vi "solar_voy_def Variant Create.vi"(8 "error in (no error)":errorcluster, 9 "Enum Names":string[](array[string]), 10 "Name":string, 11 "LVTYPE":T1) -> (0 "error out":errorcluster, 3 "Variant":variant)   [LabVIEW 2018]
doc: "This VI returns the data type of the variant. Not all data types are supported. Array of clusters are not supported."
uses:
  <vilib>/Utility/Data Type/NI_Data Type.lvlib
  <vilib>/Utility/Data Type/Type Definitions/Memory Type.ctl
  <vilib>/Utility/Data Type/Type Definitions/Memory Info.ctl
  type/solar_type Item Type.ctl
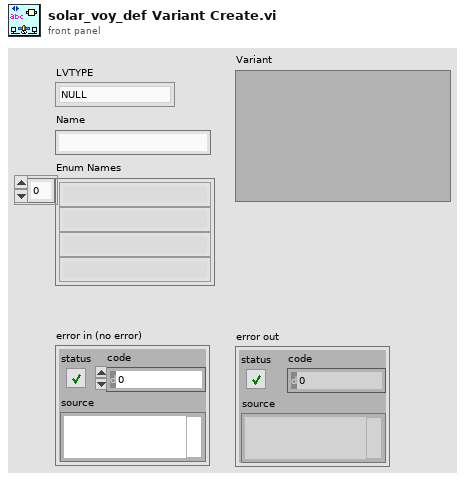
[diagram p1: front panel]
types:
  T1 = typedef "solar_type Item Type.ctl" = enum16{"NULL", "UNKNOWN", "CLUSTER", "I8", "I16", "I32", "I64", "U8", "U16", "U32", "U64", "U8_ENUM", "U16_ENUM", "U32_ENUM", "SGL", "DBL", "BOOLEAN", "STRING", "PATH", "VISA", "TAG", "TIME", "I8_1D", "I16_1D", "I32_1D", "I64_1D", "U8_1D", "U16_1D", "U32_1D", "U64_1D", "U8_ENUM_1D", "U16_ENUM_1D", "U32_ENUM_1D", "SGL_1D", "DBL_1D", "BOOLEAN_1D", "STRING_1D", "PATH_1D", "VISA_1D", "TAG_1D", "TIME_1D", "I8_2D", "I16_2D", "I32_2D", "I64_2D", "U8_2D", "U16_2D", "U32_2D", "U64_2D", "U8_ENUM_2D", "U16_ENUM_2D", "U32_ENUM_2D", "SGL_2D", "DBL_2D", "BOOLEAN_2D", "STRING_2D", "PATH_2D", "VISA_2D", "TAG_2D", "TIME_2D"}
  T2 = typedef "NI_Data Type.lvlib/Memory Info.ctl" = cluster{"Type":T3, "Size":u32}
  T3 = typedef "NI_Data Type.lvlib/Memory Type.ctl" = enum16{"Variable", "Fixed", "Bounded"}
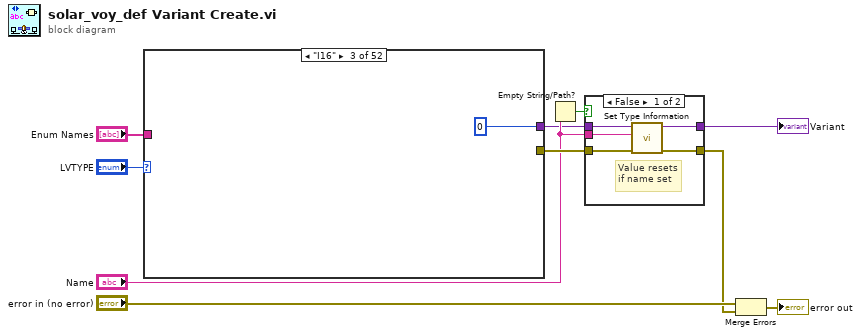
[diagram p0: block diagram]
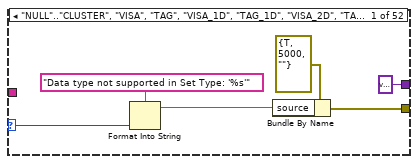
[diagram p3: hidden frame]
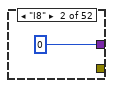
[diagram p4: hidden frame]
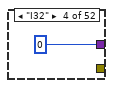
[diagram p5: hidden frame]
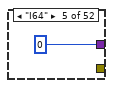
[diagram p6: hidden frame]
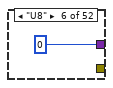
[diagram p7: hidden frame]
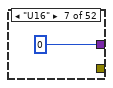
[diagram p8: hidden frame]
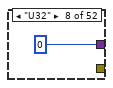
[diagram p9: hidden frame]
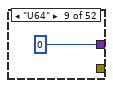
[diagram p10: hidden frame]
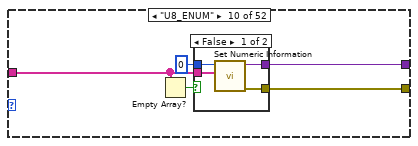
[diagram p11: hidden frame]
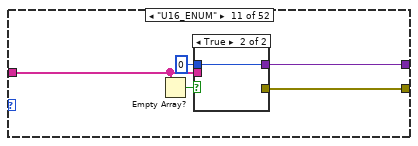
[diagram p13: hidden frame]
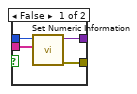
[diagram p14: hidden frame]
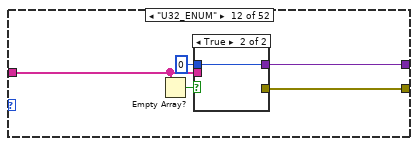
[diagram p15: hidden frame]
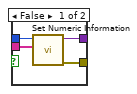
[diagram p16: hidden frame]
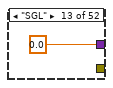
[diagram p17: hidden frame]
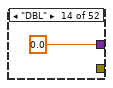
[diagram p18: hidden frame]
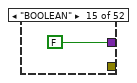
[diagram p19: hidden frame]
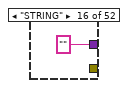
[diagram p20: hidden frame]
diagram:
  n1 = case shown="\"I16\"" "LVTYPE" {
    selector: "LVTYPE" -> [w13 _ _ _ _ _ _ _ _ _ _ _ _ _ _ _ _ _ _ _ _ _ _ _ _ _ _ _ _ _ _ _ _ _ _ _ _ _ _ _ _ _ _ _ _ _ _ _ _ _ _ _]
    tunnel: [w12 _ _ _ _ _ _ _ _ w27 w37 w47 _ _ _ _ _ _ _ _ _ _ _ _ _ _ w71 w85 w99 _ _ _ _ _ _ _ _ _ _ _ _ _ _ w128 w143 w158 _ _ _ _ _ _] -> w9
    tunnel: [variant ("Variant") i8 0 i16 0 0 i64 0 u8 0 u16 0 u32 0 u64 0 w28 w38 w48 sgl 0.0 0.0 FALSE "" path "" timestamp(0 s since 1904-01-01) i8[] [] i16[] [] i32[] [] i64[] [] u8[] [] u16[] [] u32[] [] u64[] [] w70 w84 w98 sgl[] [] dbl[] [] bool[] [] string[] [] path[] [] timestamp[] [] i8[][] [] i16[][] [] i32[][] [] i64[][] [] u8[][] [] u16[][] [] u32[][] [] u64[][] [] w127 w142 w157 sgl[][] [] dbl[][] [] bool[][] [] string[][] [] path[][] [] timestamp[][] []] -> w7
    tunnel: "Enum Names" -> [_ _ _ _ _ _ _ _ _ w26 w36 w46 _ _ _ _ _ _ _ _ _ _ _ _ _ _ w69 w83 w97 _ _ _ _ _ _ _ _ _ _ _ _ _ _ w126 w141 w156 _ _ _ _ _ _]
    frame "NULL".."CLUSTER", "VISA", "TAG", "VISA_1D", "TAG_1D", "VISA_2D", "TAG_2D" {
      n2 = Format Into String(format string="Data type not supported in Set Type: '%s'" ("source"), w13) -> (resulting string=w16:string)  [unwired: 2 in, 1 out]
      n3 = Bundle By Name(cluster=errorcluster {"status"=TRUE, "code"=5000, "source"=""} ("error out"), "source"=w16) -> (w12:errorcluster)
    }
    frame "I8" {
    }
    frame "I16" {
    }
    frame "I32" {
    }
    frame "I64" {
    }
    frame "U8" {
    }
    frame "U16" {
    }
    frame "U32" {
    }
    frame "U64" {
    }
    frame "U8_ENUM" {
      n4 = Empty Array?(array=w26) -> (empty?=w25:bool)
      n5 = case shown="False" w25 {
        tunnel: u8 0 -> [w33 w34]
        tunnel: [w32 w34] -> w28
        tunnel: [w31 _] -> w27
        tunnel: w26 -> [w30 _]
        frame False {
          n6 = call <vilib>:"Set Numeric Information.vi"("Enum Names"=w30, "Variant in"=w33) -> ("error out"=w31:errorcluster, "Variant out"=w32:variant)  [unwired: 8 in]
        }
        frame True {
        }
      }
    }
    frame "U16_ENUM" {
      n7 = Empty Array?(array=w36) -> (empty?=w35:bool)
      n8 = case shown="True" w35 {
        tunnel: u16 0 -> [w43 w44]
        tunnel: [w42 w44] -> w38
        tunnel: [w41 _] -> w37
        tunnel: w36 -> [w40 _]
        frame False {
          n9 = call <vilib>:"Set Numeric Information.vi"("Enum Names"=w40, "Variant in"=w43) -> ("error out"=w41:errorcluster, "Variant out"=w42:variant)  [unwired: 8 in]
        }
        frame True {
        }
      }
    }
    frame "U32_ENUM" {
      n10 = Empty Array?(array=w46) -> (empty?=w45:bool)
      n11 = case shown="True" w45 {
        tunnel: u32 0 -> [w53 w54]
        tunnel: [w52 w54] -> w48
        tunnel: [w51 _] -> w47
        tunnel: w46 -> [w50 _]
        frame False {
          n12 = call <vilib>:"Set Numeric Information.vi"("Enum Names"=w50, "Variant in"=w53) -> ("error out"=w51:errorcluster, "Variant out"=w52:variant)  [unwired: 8 in]
        }
        frame True {
        }
      }
    }
    frame "SGL" {
    }
    frame "DBL" {
    }
    frame "BOOLEAN" {
    }
    frame "STRING" {
    }
    frame "PATH" {
    }
    frame "TIME" {
    }
    frame "I8_1D" {
    }
    frame "I16_1D" {
    }
    frame "I32_1D" {
    }
    frame "I64_1D" {
    }
    frame "U8_1D" {
    }
    frame "U16_1D" {
    }
    frame "U32_1D" {
    }
    frame "U64_1D" {
    }
    frame "U8_ENUM_1D" {
      w74 = u8[] []
      n13 = Index Array(array=w74) -> (element=w73:u8)  [unwired: 1 in]
      n14 = Empty Array?(array=w69) -> (empty?=w77:bool)
      n15 = case shown="True" w77 {
        tunnel: w73 -> [w81 w82]
        tunnel: [w80 w82] -> w76
        tunnel: [w79 _] -> w72
        tunnel: w69 -> [w78 _]
        frame False {
          n16 = call <vilib>:"Set Numeric Information.vi"("Enum Names"=w78, "Variant in"=w81) -> ("error out"=w79:errorcluster, "Variant out"=w80:variant)  [unwired: 8 in]
        }
        frame True {
        }
      }
      n17 = call <vilib>:"Set Array Information.vi"("error in (no error)"=w72, "Array Lengths"=T2[] [{"Type"=enum."Variable", "Size"=0}], "Array Element"=w76, "Variant in"=w74) -> ("error out"=w71:errorcluster, "Variant out"=w70:variant)  [unwired: 6 in]
    }
    frame "U16_ENUM_1D" {
      w88 = u16[] []
      n18 = Index Array(array=w88) -> (element=w87:u16)  [unwired: 1 in]
      n19 = Empty Array?(array=w83) -> (empty?=w91:bool)
      n20 = case shown="True" w91 {
        tunnel: w87 -> [w95 w96]
        tunnel: [w94 w96] -> w90
        tunnel: [w93 _] -> w86
        tunnel: w83 -> [w92 _]
        frame False {
          n21 = call <vilib>:"Set Numeric Information.vi"("Enum Names"=w92, "Variant in"=w95) -> ("error out"=w93:errorcluster, "Variant out"=w94:variant)  [unwired: 8 in]
        }
        frame True {
        }
      }
      n22 = call <vilib>:"Set Array Information.vi"("error in (no error)"=w86, "Array Lengths"=T2[] [{"Type"=enum."Variable", "Size"=0}], "Array Element"=w90, "Variant in"=w88) -> ("error out"=w85:errorcluster, "Variant out"=w84:variant)  [unwired: 6 in]
    }
    frame "U32_ENUM_1D" {
      w102 = u32[] []
      n23 = Index Array(array=w102) -> (element=w101:u32)  [unwired: 1 in]
      n24 = Empty Array?(array=w97) -> (empty?=w105:bool)
      n25 = case shown="True" w105 {
        tunnel: w101 -> [w109 w110]
        tunnel: [w108 w110] -> w104
        tunnel: [w107 _] -> w100
        tunnel: w97 -> [w106 _]
        frame False {
          n26 = call <vilib>:"Set Numeric Information.vi"("Enum Names"=w106, "Variant in"=w109) -> ("error out"=w107:errorcluster, "Variant out"=w108:variant)  [unwired: 8 in]
        }
        frame True {
        }
      }
      n27 = call <vilib>:"Set Array Information.vi"("error in (no error)"=w100, "Array Lengths"=T2[] [{"Type"=enum."Variable", "Size"=0}], "Array Element"=w104, "Variant in"=w102) -> ("error out"=w99:errorcluster, "Variant out"=w98:variant)  [unwired: 6 in]
    }
    frame "SGL_1D" {
    }
    frame "DBL_1D" {
    }
    frame "BOOLEAN_1D" {
    }
    frame "STRING_1D" {
    }
    frame "PATH_1D" {
    }
    frame "TIME_1D" {
    }
    frame "I8_2D" {
    }
    frame "I16_2D" {
    }
    frame "I32_2D" {
    }
    frame "I64_2D" {
    }
    frame "U8_2D" {
    }
    frame "U16_2D" {
    }
    frame "U32_2D" {
    }
    frame "U64_2D" {
    }
    frame "U8_ENUM_2D" {
      w125 = -1 ("index (row)")
      w131 = u8[][] []
      n28 = Index Array(array=w131, index (row)=w125, index (col)=w125) -> (element=w130:u8)
      n29 = Empty Array?(array=w126) -> (empty?=w134:bool)
      n30 = case shown="True" w134 {
        tunnel: w130 -> [w138 w139]
        tunnel: [w137 w139] -> w133
        tunnel: [w136 _] -> w129
        tunnel: w126 -> [w135 _]
        frame False {
          n31 = call <vilib>:"Set Numeric Information.vi"("Enum Names"=w135, "Variant in"=w138) -> ("error out"=w136:errorcluster, "Variant out"=w137:variant)  [unwired: 8 in]
        }
        frame True {
        }
      }
      n32 = call <vilib>:"Set Array Information.vi"("error in (no error)"=w129, "Array Lengths"=T2[] [{"Type"=enum."Variable", "Size"=0}, {"Type"=enum."Variable", "Size"=0}], "Array Element"=w133, "Variant in"=w131) -> ("error out"=w128:errorcluster, "Variant out"=w127:variant)  [unwired: 6 in]
    }
    frame "U16_ENUM_2D" {
      w140 = -1 ("index (row)")
      w146 = u16[][] []
      n33 = Index Array(array=w146, index (row)=w140, index (col)=w140) -> (element=w145:u16)
      n34 = Empty Array?(array=w141) -> (empty?=w149:bool)
      n35 = case shown="True" w149 {
        tunnel: w145 -> [w153 w154]
        tunnel: [w152 w154] -> w148
        tunnel: [w151 _] -> w144
        tunnel: w141 -> [w150 _]
        frame False {
          n36 = call <vilib>:"Set Numeric Information.vi"("Enum Names"=w150, "Variant in"=w153) -> ("error out"=w151:errorcluster, "Variant out"=w152:variant)  [unwired: 8 in]
        }
        frame True {
        }
      }
      n37 = call <vilib>:"Set Array Information.vi"("error in (no error)"=w144, "Array Lengths"=T2[] [{"Type"=enum."Variable", "Size"=0}, {"Type"=enum."Variable", "Size"=0}], "Array Element"=w148, "Variant in"=w146) -> ("error out"=w143:errorcluster, "Variant out"=w142:variant)  [unwired: 6 in]
    }
    frame "U32_ENUM_2D" {
      w155 = -1 ("index (row)")
      w161 = u32[][] []
      n38 = Index Array(array=w161, index (row)=w155, index (col)=w155) -> (element=w160:u32)
      n39 = Empty Array?(array=w156) -> (empty?=w164:bool)
      n40 = case shown="True" w164 {
        tunnel: w160 -> [w168 w169]
        tunnel: [w167 w169] -> w163
        tunnel: [w166 _] -> w159
        tunnel: w156 -> [w165 _]
        frame False {
          n41 = call <vilib>:"Set Numeric Information.vi"("Enum Names"=w165, "Variant in"=w168) -> ("error out"=w166:errorcluster, "Variant out"=w167:variant)  [unwired: 8 in]
        }
        frame True {
        }
      }
      n42 = call <vilib>:"Set Array Information.vi"("error in (no error)"=w159, "Array Lengths"=T2[] [{"Type"=enum."Variable", "Size"=0}, {"Type"=enum."Variable", "Size"=0}], "Array Element"=w163, "Variant in"=w161) -> ("error out"=w158:errorcluster, "Variant out"=w157:variant)  [unwired: 6 in]
    }
    frame "SGL_2D" {
    }
    frame "DBL_2D" {
    }
    frame "BOOLEAN_2D" {
    }
    frame "STRING_2D" {
    }
    frame "PATH_2D" {
    }
    frame "TIME_2D" {
    }
  }
  n43 = Empty String/Path?(string/path="Name") -> (empty?=w5:bool)
  n44 = case shown="False" w5 {
    tunnel: [w177 w181] -> w2
    tunnel: w9 -> [w178 w181]
    tunnel: "Name" -> [w179 _]
    tunnel: w7 -> [w180 w182]
    tunnel: [w176 w182] -> w6
    frame False {
      # "Value resets\nif name set"
      n45 = call <vilib>:"Set Type Information.vi"("error in (no error)"=w178, "Name"=w179, "Variant in"=w180) -> ("error out"=w177:errorcluster, "Variant out"=w176:variant)  [unwired: 7 in]
    }
    frame True {
    }
  }
  "Variant" <- w6
  n46 = Merge Errors("error in (no error)", w2) -> (→"error out":errorcluster)
